vi "enqueue.vi"(6 "priority (f)":bool, 8 "error in (no error)":errorcluster, 9 "data":variant, 10 "cmd":T1, 11 "comic_crawler in":refnum<class "comic_crawler.lvclass">) -> (0 "error out":errorcluster, 3 "comic_crawler out":refnum<class "comic_crawler.lvclass">)   [LabVIEW 2024, in "comic_crawler.lvclass"]
uses:
  comic_crawler.lvclass
  comic_crawler.lvclass/comic_crawler.ctl
  daemon.states--enum.ctl
  queue.message--cluster.ctl
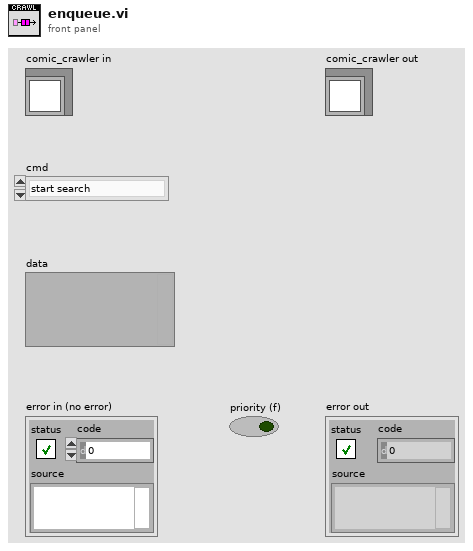
[diagram p1: front panel]
types:
  T1 = typedef "comic_crawler.lvclass/daemon.states--enum.ctl" = enum16{"start search", "waiting", "running", "stop search", "wait", "shut down"}
  T2 = typedef "comic_crawler.lvclass/queue.message--cluster.ctl" = cluster{"cmd":T1, "data":variant}
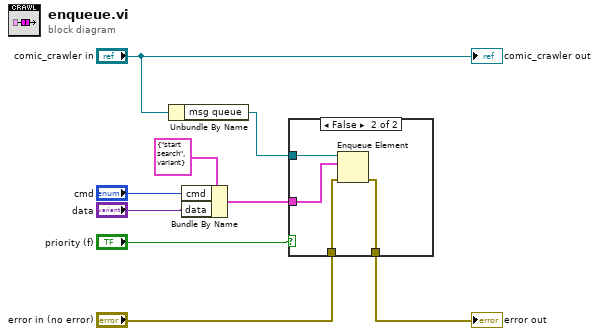
[diagram p0: block diagram]
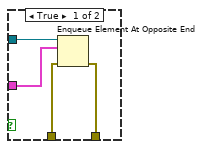
[diagram p2: hidden frame]
diagram:
  n1 = Unbundle By Name("comic_crawler in") -> ("msg queue"=w8:refnum<queue>)
  n2 = Bundle By Name(cluster=T2 {"cmd"=enum."start search", "data"=variant} ("message"), "cmd"="cmd", "data"="data") -> (w3:T2)
  n3 = case shown="False" "priority (f)" {
    tunnel: w8 -> [w13 w17]
    tunnel: "error in (no error)" -> [w12 w16]
    tunnel: [w11 w15] -> w6
    tunnel: w3 -> [w10 w14]
    frame True {
      n4 = Enqueue Element At Opposite End(queue=w13, element=w10, error in (no error)=w12) -> (error out=w11:errorcluster)  [unwired: 1 in, 2 out]
    }
    frame False {
      n5 = Enqueue Element(queue=w17, element=w14, error in (no error)=w16) -> (error out=w15:errorcluster)  [unwired: 1 in, 2 out]
    }
  }
  "error out" <- w6
  "comic_crawler out" <- "comic_crawler in"
